vi "Create_Alias_File.vi"(8 "error in (no error)":errorcluster, 11 "AB_Application in":refnum<class "AB_Application.lvclass">) -> (0 "error out":errorcluster, 3 "AB_Application out":refnum<class "AB_Application.lvclass">)   [LabVIEW 2020, in "AB_Application.lvclass"]
uses:
  <vilib>/AppBuilder/AB_Classes/Application/AB_Application.lvclass
  e:/builds/penguin/labview/branches/2020/dev/dist/vi.lib/AppBuilder/AB_Classes/TargetFile/AB_Targetfile.lvclass
  e:/builds/penguin/labview/branches/2020/dev/dist/vi.lib/AppBuilder/AB_Classes/Build/AB_Build.lvclass
  <vilib>/AppBuilder/AB_Classes/Application/AB_Application.lvclass/AB_Application.ctl
  <vilib>/Utility/config.llb/Write Key (String).vi
  <resource>/Framework/Providers/Common/provcom_StringGlobals.vi
  <vilib>/Utility/config.llb/NI_LVConfig.lvlib
  <vilib>/AppBuilder/AB_Classes/Build/AB_Build.lvclass
  <vilib>/AppBuilder/AB_Classes/TargetFile/AB_Targetfile.lvclass
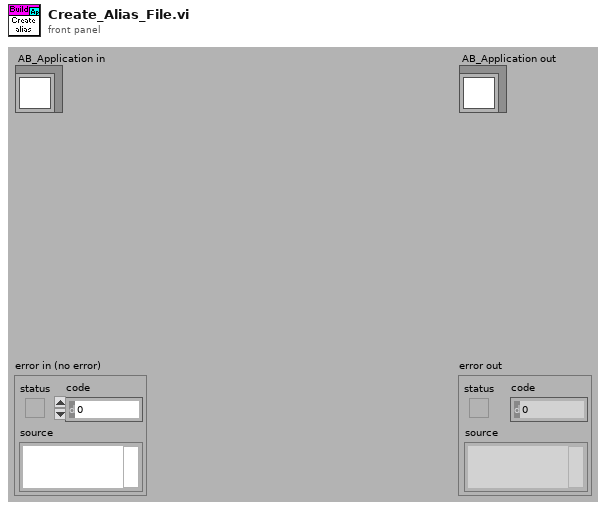
[diagram p1: front panel]
types:
  T1 = typedef "AB_Targetfile.ctl" = cluster{"targetfileName":string, "targetfileGUID":string, "enableDebugging":bool, "versionInfo":cluster{"productName":string, "legalCopyright":string, "companyName":string, "internalName":string, "fileDescription":string}, "eng_consolidatedTypeInfo":string, "fastFileFormat":bool, "eng_LEIFBuildData":u32, "versionIndependent":bool}
  T2 = typedef "AB_Build.ctl" = cluster{"buildSpecName":string, "buildSpecDescription":string, "destinations":refnum<class "AB_Destination.lvclass">[], "exclusionOption":T3, "defaultLanguage":string, "supportedLanguages":string[], "excludedDirectories":path[], "buildContext":refnum<vi>, "buildObject":T4, "preview":bool, "programatic":bool, "progressBarEvents":T5, "userLog_Path":path, "preActionID":string, "preAction_Path":path, "postActionID":string, "postAction_Path":path, "eng_checkForBrokenVIs?":bool, "eng_verboseLinkerErrors?":bool, "localDest_Path":path, "targetDest_Path":path, "removeVIObject":u16, "cache":refnum<class "PreviewCache.lvclass">, "use cache":bool, "previewCache_ID":string, "buildCache_ID":string, "eng_TempLocalDest_Path":path, "eng_collectDependencies?":bool, "versionInfo":cluster{"buildVersion":cluster{"major":u16, "minor":u16, "patch":u16, "build":u16}, "autoIncrement":bool}, "eng_enableVIChecksums":bool}
  T3 = typedef "AB_Exclusion_Option.ctl" = cluster{"typedefs":bool, "polymorphicVIs":bool, "unusedLibraryItems":bool, "modifyLibraryFile":bool, "edit-timeDependencies":bool, "inlineVIs":bool, "dependent PPLs":bool, "dependent DLLs":bool}
  T4 = typedef "ItemRef.ctl" = u64
  T5 = typedef "provcom_ProgressBar_Events.ctl" = cluster{"newJob":refnum<user-event>, "newItem":refnum<user-event>, "errorMsg":T6, "cancel":refnum<user-event>}
  T6 = typedef "mxLvBuildError.ctl" = refnum<user-event>
  T7 = typedef "NI_LVConfig.lvlib/Config Data RefNum.ctl" = refnum<k1>
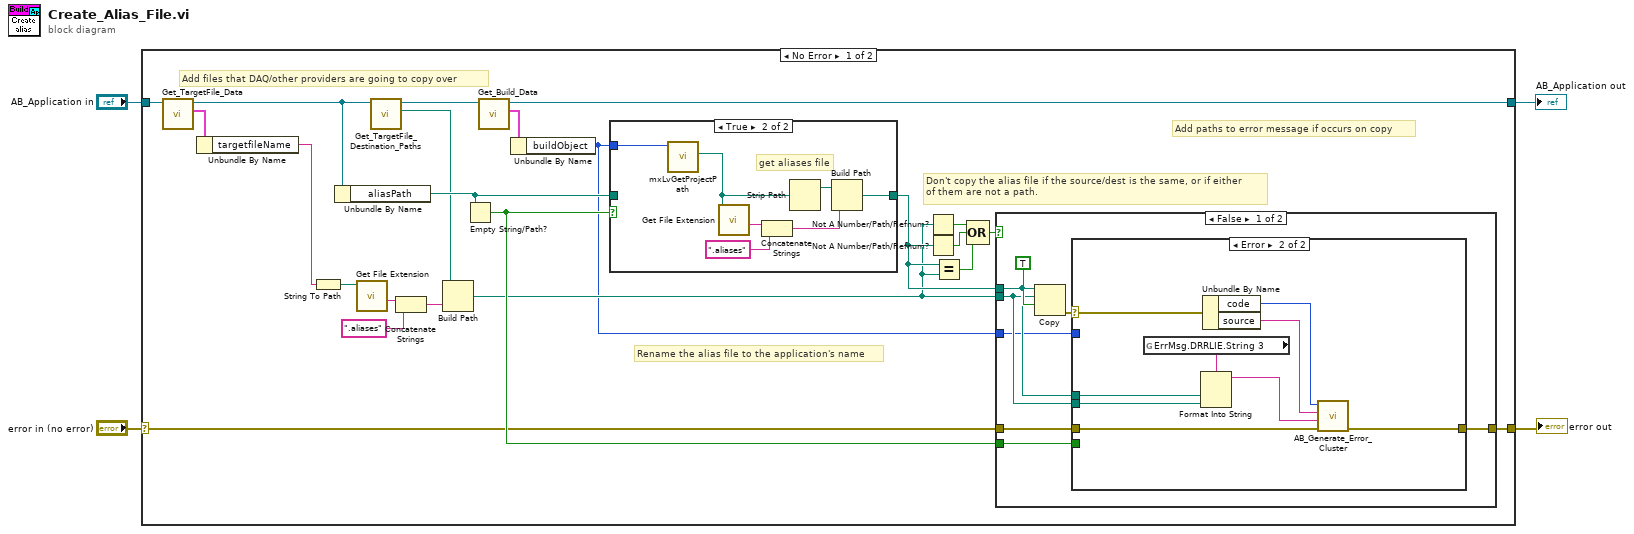
[diagram p0: block diagram]
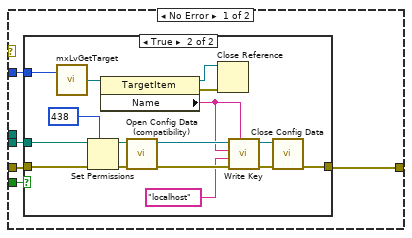
[diagram p2: hidden frame]
diagram:
  n1 = case shown="No Error" "error in (no error)" {
    selector: "error in (no error)" -> [w25 w77]
    tunnel: [w22 w77] -> w3
    tunnel: [w10 w76] -> w1
    tunnel: "AB_Application in" -> [w8 w76]
    frame No Error {
      # "Don't copy the alias file if the source/dest is the same, or if either\nof them are not a path."
      # "Add paths to error message if occurs on copy"
      # "Rename the alias file to the application's name"
      # "Add files that DAQ/other providers are going to copy over"
      n2 = call <vilib>:"Get_TargetFile_Data.vi"("AB_Targetfile in"=w8) -> ("data"=w7:T1, "AB_Targetfile out"=w6:refnum<class "AB_Application.lvclass">)  [unwired: 8 in, 1 out]
      n3 = Unbundle By Name(w7) -> ("targetfileName"=w5:string)
      n4 = String To Path(string=w5) -> (path=w14:path)
      n5 = Unbundle By Name(w6) -> ("aliasPath"=w27:path)
      n6 = call <vilib>:"Get File Extension.vi"("file"=w14) -> ("filename without extension"=w17:string)  [unwired: 1 in, 9 out]
      n7 = call <vilib>:"Get_TargetFile_Destination_Paths.vi"("AB_Targetfile in"=w6) -> ("destination path"=w13:path, "AB_Targetfile out"=w11:refnum<class "AB_Application.lvclass">)  [unwired: 1 in, 8 out]
      n8 = Concatenate Strings(w17, ".aliases" ("string")) -> (w16:string)
      n9 = Build Path(base path=w13, name or relative path=w16) -> (appended path=w15:path)
      n10 = Empty String/Path?(string/path=w27) -> (empty?=w26:bool)
      n11 = call <vilib>:"Get_Build_Data.vi"("Class in"=w11) -> ("data"=w12:T2, "Class out"=w10:refnum<class "AB_Application.lvclass">)  [unwired: 1 in, 8 out]
      n12 = Unbundle By Name(w12) -> ("buildObject"=w9:T4)
      n13 = case shown="True" w26 {
        tunnel: [w68 w71] -> w24
        tunnel: w27 -> [w68 _]
        tunnel: w9 -> [_ w69]
        frame False {
          # "If the alias isn't Project.aliases, then it's an ItemID\nfor a specified configuration file, so copy that file\nto where the INI should be."
        }
        frame True {
          # "get aliases file"
          n14 = call <resource>:"mxLvGetProjectPath.vi"("Item"=w69) -> ("Project Path"=w70:path)  [unwired: 1 in, 9 out]
          n15 = call <vilib>:"Get File Extension.vi"("file"=w70) -> ("filename without extension"=w74:string)  [unwired: 1 in, 9 out]
          n16 = Concatenate Strings(w74, ".aliases" ("string")) -> (w73:string)
          n17 = Strip Path(path=w70) -> (stripped path=w72:path)  [unwired: 1 out]
          n18 = Build Path(base path=w72, name or relative path=w73) -> (appended path=w71:path)
        }
      }
      n19 = Not A Number/Path/Refnum?(number/path/refnum=w15) -> (NaN/Path/Refnum?=w21:bool)
      n20 = Not A Number/Path/Refnum?(number/path/refnum=w24) -> (NaN/Path/Refnum?=w20:bool)
      n21 = Equal?(x=w24, y=w15) -> (x = y?=w18:bool)
      n22 = Compound Arithmetic op=OR(w21, w20, w18) -> (w19:bool)
      n23 = case shown="False" w19 {
        tunnel: w24 -> [w33 _]
        tunnel: w15 -> [w32 _]
        tunnel: [w31 w67] -> w22
        tunnel: w25 -> [w30 w67]
        tunnel: w26 -> [w29 _]
        tunnel: w9 -> [w28 _]
        frame False {
          n24 = Copy(9:TRUE ("overwrite (F)"), 10:w32, 11:w33) -> (0:w34:errorcluster)  [unwired: 1 in, 3 out]
          n25 = case shown="Error" w34 {
            selector: w34 -> [_ w61]
            tunnel: w33 -> [_ w64]
            tunnel: w32 -> [w38 w63]
            tunnel: [w39 w60] -> w31
            tunnel: w30 -> [w40 w59]
            tunnel: w29 -> [w37 _]
            tunnel: w28 -> [w36 _]
            frame No Error {
              n26 = case shown="True" w37 {
                tunnel: w40 -> [w41 w49]
                tunnel: [w41 w48] -> w39
                tunnel: w38 -> [_ w47]
                tunnel: w36 -> [_ w45]
                frame False {
                }
                frame True {
                  n27 = call <resource>:"mxLvGetTarget.vi"("Item"=w45) -> ("Target"=w46:refnum<vi>)  [unwired: 1 in, 2 out]
                  n28 = Set Permissions(7:i16 438 ("permissions"), 8:w49, 11:w47) -> (0:w57:errorcluster, 3:w56:path)  [unwired: 2 out]
                  n29 = property class="TargetItem"(reference=w46) -> (reference out=w42:refnum<vi>, error out=w43:errorcluster, "Name"=w44:string)  [unwired: 1 in]
                  n30 = call <vilib>:"Open Config Data (compatibility).vi"("error in (no error)"=w57, "configuration file path"=w56) -> ("error out"=w53:errorcluster, "refnum"=w50:T7)  [unwired: 7 in, 1 out]
                  n31 = Close Reference(reference=w42, error in (no error)=w43) -> ()  [unwired: 1 out]
                  n32 = call-poly <vilib>:"Write Key.vi"("section"=w44, "error in (no error)"=w53, "value"="localhost" ("key"), "key"=w44, "refnum"=w50) -> ("error out"=w54:errorcluster, "refnum out"=w51:T7)  [unwired: 1 in, 4 out]
                  n33 = call <vilib>:"Close Config Data.vi"("error in (no error)"=w54, "refnum"=w51) -> ("error out"=w48:errorcluster)  [unwired: 1 in, 8 out]
                }
              }
            }
            frame Error {
              n34 = global read "provcom_StringGlobals.vi" "ErrMsg.DRRLIE.String 3"() -> (w58:string)
              n35 = Format Into String(format string=w58, w64, w63) -> (resulting string=w62:string)  [unwired: 2 in, 1 out]
              n36 = Unbundle By Name(w61) -> ("code"=w66:i32, "source"=w65:string)
              n37 = call <vilib>:"AB_Generate_Error_Cluster.vi"("error in (no error)"=w59, "Additional Message"=w62, "source"=w65, "Code"=w66) -> ("error out"=w60:errorcluster)  [unwired: 7 out]
            }
          }
        }
        frame True {
        }
      }
    }
    frame Error {
    }
  }
  "error out" <- w3
  "AB_Application out" <- w1
